vi "Launch LV Instance.vi"(8 "error in (no error)":errorcluster, 9 "Show":bool=TRUE, 10 "Port":i32=4545, 11 "BuildWorker Controller in":refnum<class "BuildWorker Controller.lvclass">) -> (0 "error out":errorcluster, 3 "BuildWorker Controller out":refnum<class "BuildWorker Controller.lvclass">)   [LabVIEW 2017, in "BuildWorker Controller.lvlib" / "BuildWorker Controller.lvclass"]
uses:
  BuildWorker Controller.lvclass
  BuildWorker Controller.lvclass/BuildWorker Controller.ctl
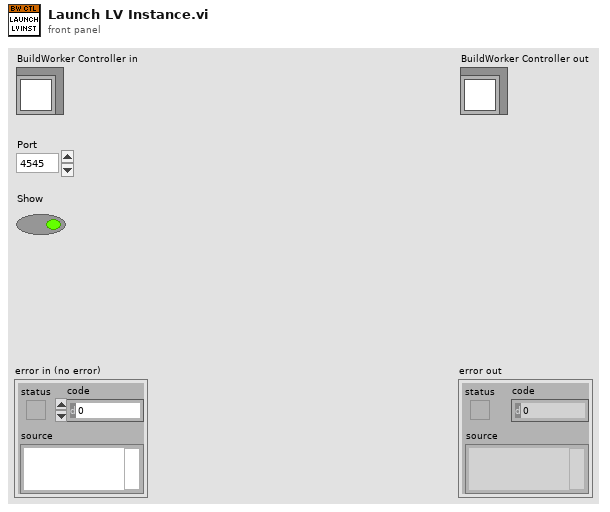
[diagram p1: front panel]
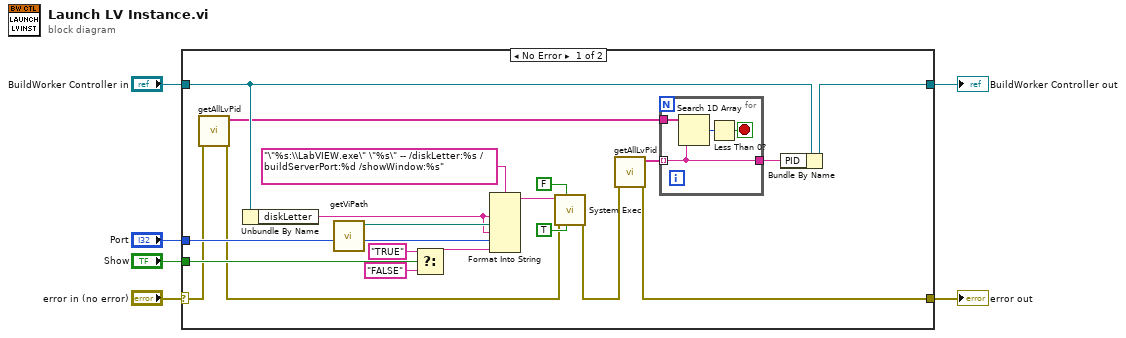
[diagram p0: block diagram]
diagram:
  n1 = case shown="No Error" "error in (no error)" {
    selector: "error in (no error)" -> [w13 w32]
    tunnel: [w11 w32] -> w5
    tunnel: [w8 w31] -> w3
    tunnel: "BuildWorker Controller in" -> [w26 w31]
    tunnel: "Port" -> [w22 _]
    tunnel: "Show" -> [w21 _]
    frame No Error {
      n2 = call "getAllLvPid.vi"("error in (no error)"=w13) -> ("error out"=w14:errorcluster, "PIDs"=w10:string[])  [unwired: 9 in]
      n3 = Unbundle By Name(w26) -> ("diskLetter"=w23:string)
      n4 = call "getViPath.vi"() -> ("VI Path"=w24:path)  [unwired: 11 in]
      n5 = Select(t="TRUE", s=w21, f="FALSE") -> (s? t:f=w18:string)
      n6 = Format Into String(format string="\"%s:\\LabVIEW.exe\" \"%s\" -- /diskLetter:%s /buildServerPort:%d /showWindow:%s", w23, w24, w23, w22, w18) -> (resulting string=w17:string)  [unwired: 2 in, 1 out]
      n7 = call <vilib>:"System Exec.vi"("run minimized? (F)"=TRUE, "wait until completion? (T)"=FALSE, "error in (no error)"=w14, "command line"=w17) -> ("error out"=w12:errorcluster)  [unwired: 4 in, 3 out]
      n8 = call "getAllLvPid.vi"("error in (no error)"=w12) -> ("error out"=w11:errorcluster, "PIDs"=w9:string[])  [unwired: 9 in]
      n9 = for {
        tunnel: w10 -> [w30]
        tunnel: w9 -> [w27] mode=indexing
        tunnel: [w27] -> w7
        stop <- w28 stop-if-true
        n10 = Search 1D Array(1D array=w30, element=w27) -> (index of element=w29:i32)  [unwired: 1 in]
        n11 = Less Than 0?(x=w29) -> (x < 0?=w28:bool)
      }
      n12 = Bundle By Name(cluster=w26, "PID"=w7) -> (w8:refnum<class "BuildWorker Controller.lvclass">)
    }
    frame Error {
    }
  }
  "error out" <- w5
  "BuildWorker Controller out" <- w3
